vi "Send Query.vi"(8 "error in (no error)":errorcluster, 9 "Bytes Count":u32=1024, 10 "write buffer":string, 11 "VISA resource name":refnum<visa-resource-name>) -> (0 "error out":errorcluster, 2 "read buffer":string, 3 "VISA resource name out":refnum<visa-resource-name>)   [LabVIEW 2017, in "Agilent PSG MXG Series.lvlib"]
uses:
  Agilent PSG MXG Series.lvlib
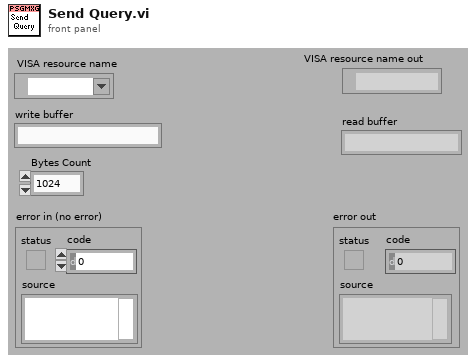
[diagram p1: front panel]
types:
  T1 = typedef "Semaphore RefNum" = refnum<k1>
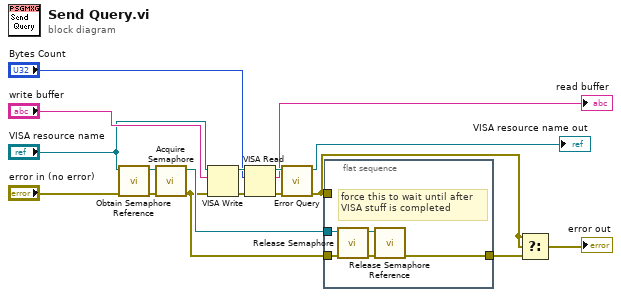
[diagram p0: block diagram]
diagram:
  n1 = call <vilib>:"Obtain Semaphore Reference.vi"("error in (no error)"="error in (no error)", "name (unnamed)"="VISA resource name") -> ("error out"=w8:errorcluster, "semaphore"=w9:T1)  [unwired: 1 in, 3 out]
  n2 = call <vilib>:"Acquire Semaphore.vi"("error in (no error)"=w8, "semaphore"=w9) -> ("error out"=w2:errorcluster, "semaphore out"=w6:T1)  [unwired: 1 in, 3 out]
  n3 = VISA Write(VISA resource name="VISA resource name", write buffer="write buffer", error in (no error)=w2) -> (VISA resource name out=w17:refnum<visa-resource-name>, error out=w15:errorcluster)  [unwired: 1 out]
  n4 = VISA Read(VISA resource name=w17, byte count="Bytes Count", error in (no error)=w15) -> (VISA resource name out=w13:refnum<visa-resource-name>, read buffer=→"read buffer":string, error out=w12:errorcluster)  [unwired: 1 out]
  n5 = call "Error Query.vi"("error in (no error)"=w12, "VISA resource name"=w13) -> ("error out"=w1:errorcluster, "VISA resource name out"=→"VISA resource name out":refnum<visa-resource-name>)  [unwired: 8 out]
  n6 = flat-sequence {
    tunnel: w6 -> [w22]
    tunnel: [w19] -> w3
    tunnel: w2 -> [w18]
    tunnel: w1 -> [_]
    frame #0 {
      # "force this to wait until after \nVISA stuff is completed"
      n7 = call <vilib>:"Release Semaphore.vi"("error in (no error)"=w18, "semaphore"=w22) -> ("error out"=w20:errorcluster, "semaphore out"=w21:T1)  [unwired: 4 out]
      n8 = call <vilib>:"Release Semaphore Reference.vi"("error in (no error)"=w20, "semaphore"=w21) -> ("error out"=w19:errorcluster)  [unwired: 9 out]
    }
  }
  n9 = Select(t=w1, s=w1, f=w3) -> (s? t:f=→"error out":errorcluster)
